vi "Initialize.vi"(8 "error in (no error)":errorcluster, 11 "socket SUB in":refnum<class "socket SUB.lvclass">) -> (0 "error out":errorcluster, 3 "socket SUB out":refnum<class "socket SUB.lvclass">)   [LabVIEW 2018, in "socket SUB.lvclass"]
uses:
  socket SUB.lvclass
  C:/Users/orlando/Documents/Orlando/communication-manager/communication-manager/Socket/Socket.lvclass
  Socket/Socket.lvclass
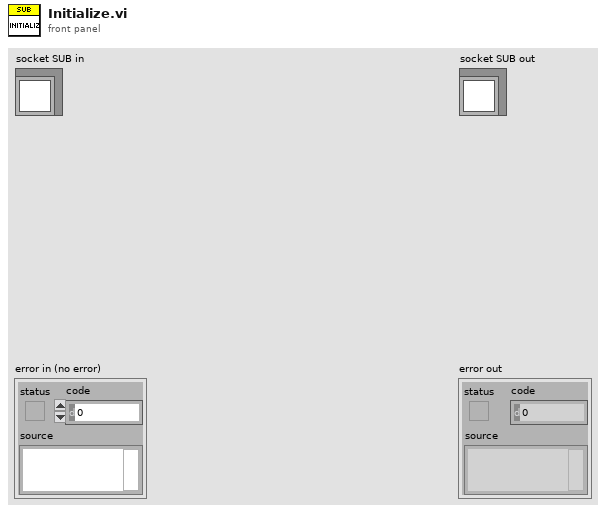
[diagram p1: front panel]
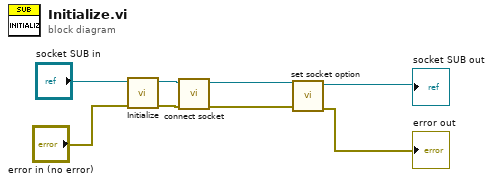
[diagram p0: block diagram]
diagram:
  n1 = call-parent "Initialize.vi"("error in (no error)"="error in (no error)", "Socket in"="socket SUB in") -> ("error out"=w5:errorcluster, "Socket out"=w6:refnum<class "socket SUB.lvclass">)  [unwired: 8 in]
  n2 = call "connect socket.vi"("error in (no error)"=w5, "Socket in"=w6) -> ("error out"=w1:errorcluster, "Socket out"=w2:refnum<class "socket SUB.lvclass">)  [unwired: 8 in]
  n3 = call "set socket option.vi"("error in (no error)"=w1, "Socket2 in"=w2) -> ("error out"=→"error out":errorcluster, "Socket2 out"=→"socket SUB out":refnum<class "socket SUB.lvclass">)  [unwired: 8 in]
